vi "Trace Update Trace Points.vi"(7 "index":i32, 9 "Status of previous command":T1, 10 "New Point":cluster{dbl, i32}, 11 "Array in":cluster{"Tracings":cluster{dbl, dbl}[]}[](array[cluster])) -> (3 "Array out":cluster{"Tracings":cluster{dbl, dbl}[]}[](array[cluster]))   [LabVIEW 2025]
uses:
  <vilib>/Rock Robotics/WPI/Framework/Completion Status.ctl
panel:
  in  "History Size":i32=1000
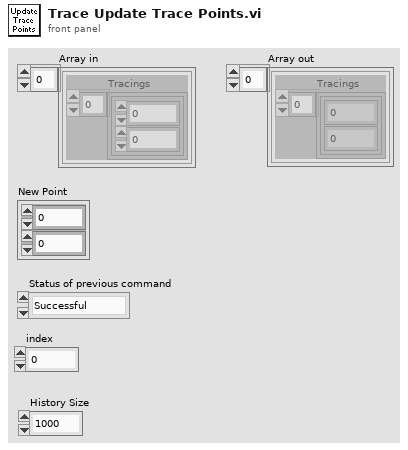
[diagram p1: front panel]
types:
  T1 = typedef "Completion Status.ctl" = enum16{"Successful", "Aborted", "Incomplete"}
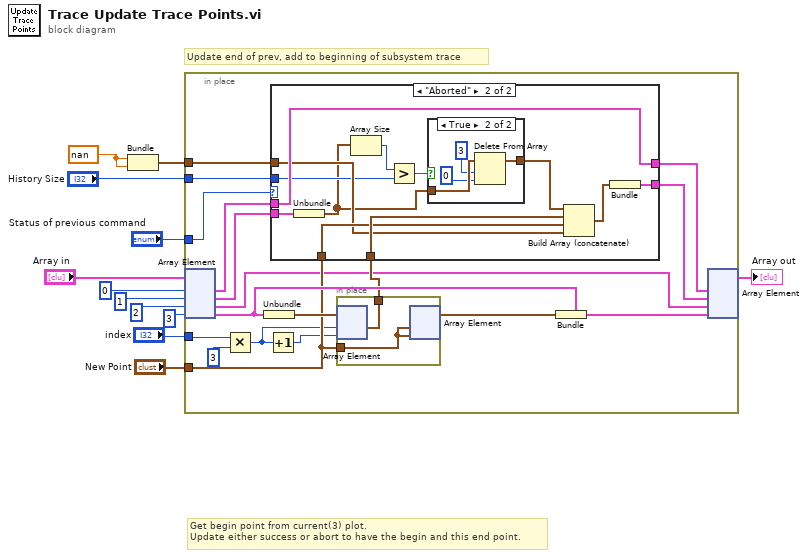
[diagram p0: block diagram]
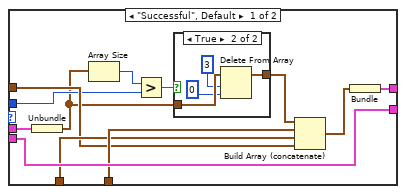
[diagram p2: hidden frame]
diagram:
  w4 = nan
  # "Get begin point from current(3) plot.\nUpdate either success or abort to have the begin and this end point."
  # "Update end of prev, add to beginning of subsystem trace"
  n1 = Bundle(w4, w4) -> (w3:cluster{dbl, dbl})  [unwired: 1 in]
  n2 = in-place {
    in-place-border: "index" -> [w29]
    in-place-border: "New Point" -> [w20]
    in-place-border: "Status of previous command" -> [w24]
    in-place-border: w3 -> [w14]
    in-place-border: "History Size" -> [w13]
    n3 = in-place-array #1("Array in", 0, 1, 2, 3) -> (w23:cluster{"Tracings":cluster{dbl, dbl}[]}, w22:cluster{"Tracings":cluster{dbl, dbl}[]}, w17:cluster{"Tracings":cluster{dbl, dbl}[]}, w28:cluster{"Tracings":cluster{dbl, dbl}[]})
    n4 = Multiply(x=w29, y=3) -> (x*y=w16:i32)
    n5 = Unbundle(w28) -> ("Tracings"=w25:cluster{dbl, dbl}[])
    n6 = Increment(x=w16) -> (x+1=w15:i32)
    n7 = in-place {
      in-place-border: w20 -> [w66]
      in-place-border: [w65] -> w21
      n8 = in-place-array #2(w25, w16, w15) -> (w65:cluster{dbl, dbl})  [unwired: 1 out]
      n9 = in-place-array #2(w66, w66) -> (w26:cluster{dbl, dbl}[])  [unwired: 2 out]
    }
    n10 = case shown="\"Aborted\"" w24 {
      tunnel: w23 -> [w42 w57]
      tunnel: w22 -> [w40 w59]
      tunnel: w21 -> [w39 w55]
      tunnel: w20 -> [w38 w54]
      tunnel: [w40 w58] -> w18
      tunnel: [w41 w57] -> w19
      tunnel: w14 -> [w37 w53]
      tunnel: w13 -> [w36 w52]
      frame "Successful", Default {
        n11 = Unbundle(w42) -> ("Tracings"=w34:cluster{dbl, dbl}[])
        n12 = Array Size(array=w34) -> (size(s)=w33:i32)
        n13 = Greater?(x=w33, y=w36) -> (0:w35:bool)
        n14 = case shown="True" w35 {
          tunnel: w34 -> [w43 w47]
          tunnel: [w43 w44] -> w31
          frame False {
          }
          frame True {
            n15 = Delete From Array(array=w47, length=3, index=0) -> (array with subset deleted=w44:cluster{dbl, dbl}[])  [unwired: 1 out]
          }
        }
        n16 = Build Array (concatenate)(w31, w39, w38, w37) -> (w32:cluster{dbl, dbl}[])
        n17 = Bundle(w32) -> (w41:cluster{cluster{dbl, dbl}[]})  [unwired: 1 in]
      }
      frame "Aborted" {
        n18 = Unbundle(w59) -> ("Tracings"=w49:cluster{dbl, dbl}[])
        n19 = Array Size(array=w49) -> (size(s)=w51:i32)
        n20 = Greater?(x=w51, y=w52) -> (0:w50:bool)
        n21 = case shown="True" w50 {
          tunnel: w49 -> [w60 w64]
          tunnel: [w60 w61] -> w48
          frame False {
          }
          frame True {
            n22 = Delete From Array(array=w64, length=3, index=0) -> (array with subset deleted=w61:cluster{dbl, dbl}[])  [unwired: 1 out]
          }
        }
        n23 = Build Array (concatenate)(w48, w55, w54, w53) -> (w56:cluster{dbl, dbl}[])
        n24 = Bundle(w56) -> (w58:cluster{cluster{dbl, dbl}[]})  [unwired: 1 in]
      }
    }
    n25 = Bundle(cluster=w28, "Tracings"=w26) -> (w27:cluster{"Tracings":cluster{dbl, dbl}[]})
    n26 = in-place-array #1(w19, w18, w17, w27) -> (→"Array out":cluster{"Tracings":cluster{dbl, dbl}[]}[])  [unwired: 4 out]
  }
